vi "MeasurementsFFT.vi"(10 "Left Lobe EEG":dynamicdata(waveform), 11 "Control in":refnum<vi>) -> (2 "Spectrum Out":cluster{"f0":dbl, "df":dbl, "S(f)":dbl[]}, 3 "Frequency Measurements":T1)   [LabVIEW 2019]
uses:
  <vilib>/addons/Biomedical/Biosignal Measurements/EEG/subVIs/bmt_EEG Frequency-domain Measures.ctl
  <vilib>/addons/Biomedical/Controls/Biosignal/Biosignal Spectrum/Biosignal Spectrum.xctl
  <vilib>/addons/Biomedical/Biosignal Measurements/EEG/subVIs/bmt_EEG FFT Settings.ctl
  <vilib>/addons/Biomedical/Biosignal Measurements/EEG/subVIs/bmt_EEG Frequency Bands.ctl
  <vilib>/addons/Biomedical/Biosignal Measurements/EEG/EEG FFT Spectrum (Waveform).vi
  <vilib>/addons/Biomedical/NI_BMTK_Measurements.lvlib
  <vilib>/addons/Biomedical/NI_BMTK_Controls.lvlib
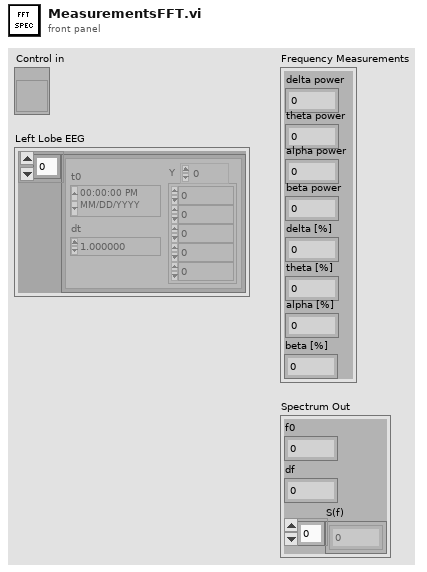
[diagram p1: front panel]
types:
  T1 = typedef "NI_BMTK_Measurements.lvlib/bmt_EEG Frequency-domain Measures.ctl" = cluster{"delta power":dbl, "theta power":dbl, "alpha power":dbl, "beta power":dbl, "delta [%]":dbl, "theta [%]":dbl, "alpha [%]":dbl, "beta [%]":dbl}
  T2 = typedef "NI_BMTK_Measurements.lvlib/bmt_EEG FFT Settings.ctl" = cluster{"window settings":cluster{"window":u16, "length":i32, "overlap [%]":dbl}, "frequency bands":T3, "dB on? (F)":bool, "frequency bins":i32}
  T3 = typedef "NI_BMTK_Measurements.lvlib/bmt_EEG Frequency Bands.ctl" = cluster{"delta high":dbl, "delta low":dbl, "theta high":dbl, "theta low":dbl, "alpha high":dbl, "alpha low":dbl, "beta high":dbl, "beta low":dbl}
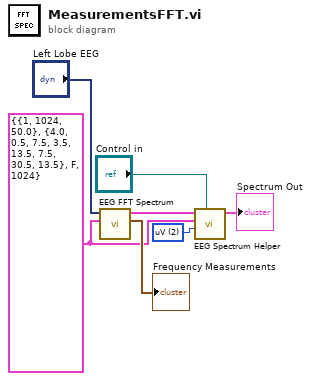
[diagram p0: block diagram]
diagram:
  w5 = T2 {"window settings"={"window"=1, "length"=1024, "overlap [%]"=50.0}, "frequency bands"={"delta high"=4.0, "delta low"=0.5, "theta high"=7.5, "theta low"=3.5, "alpha high"=13.5, "alpha low"=7.5, "beta high"=30.5, "beta low"=13.5}, "dB on? (F)"=FALSE, "frequency bins"=1024} ("FFT setttings")
  w1 = u16 2 items=["V", "mV", "uV"] ("RR unit")
  n1 = call-poly <vilib>:"EEG FFT Spectrum.vi"("FFT setttings"=w5, "EEG"="Left Lobe EEG") -> ("frequency measurements"=→"Frequency Measurements":T1, "FFT spectrum"=w4:cluster{"f0":dbl, "df":dbl, "S(f)":dbl[]})  [unwired: 7 in, 1 out]
  n2 = call <vilib>:"EEG Spectrum Helper.vi"("EEG spectrum"="Control in", "EEG unit"=w1, "FFT settings"=w5, "spectrum in"=w4) -> ("spectrum out"=→"Spectrum Out":cluster{"f0":dbl, "df":dbl, "S(f)":dbl[]})  [unwired: 6 in, 1 out]
